vi "Set TDD Flag.vi"(8 "error in":errorcluster, 10 "TDD Mode (T=Run Tests)":bool=TRUE) -> (0 "error out":errorcluster)   [LabVIEW 2014]
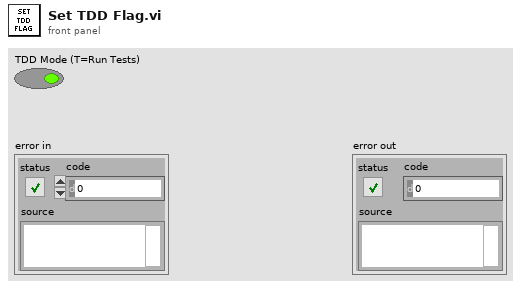
[diagram p1: front panel]
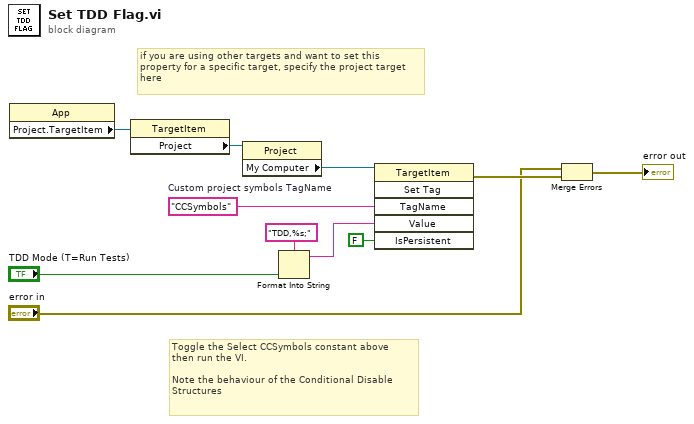
[diagram p0: block diagram]
diagram:
  w6 = "CCSymbols"  # Custom project symbols TagName
  # "if you are using other targets and want to set this property for a specific target, specify the project target here"
  # "Toggle the Select CCSymbols constant above\nthen run the VI.\n\nNote the behaviour of the Conditional Disable \nStructures"
  n1 = property class="App"() -> ("Project.TargetItem"=w2:refnum<vi>)  [unwired: 2 in, 2 out]
  n2 = property class="TargetItem"(reference=w2) -> ("Project"=w1:refnum<vi>)  [unwired: 1 in, 2 out]
  n3 = property class="Project"(reference=w1) -> ("My Computer"=w11:refnum<vi>)  [unwired: 1 in, 2 out]
  n4 = Format Into String(format string="TDD,%s;", "TDD Mode (T=Run Tests)") -> (resulting string=w9:string)  [unwired: 2 in, 1 out]
  n5 = invoke class="TargetItem" method="Set Tag"(reference=w11, "TagName"=w6, "Value"=w9, "IsPersistent"=FALSE ("Is Persistent")) -> (error out=w7:errorcluster)  [unwired: 2 in, 5 out]
  n6 = Merge Errors("error in", w7) -> (→"error out":errorcluster)
